vi "Handle.vi"(7 "Event jettl in":refnum<class "Event Actor.lvclass">, 11 "Teardown State in":refnum<class "Teardown State.lvclass">) -> (2 "Destroy?":bool, 5 "Event jettl out":refnum<class "Event Actor.lvclass">)   [LabVIEW 2021, in "jettl.lvlib" / "Base Event jettl.lvlib" / "Teardown State.lvclass"]
uses:
  Teardown State.lvclass
  Actor/Event Actor/Event Actor.lvclass
  Teardown State.lvclass/Teardown State.ctl
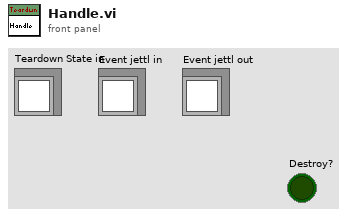
[diagram p1: front panel]
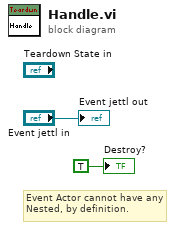
[diagram p0: block diagram]
diagram:
  # "Event Actor cannot have any Nested, by definition."
  "Destroy?" <- TRUE ("Destroy?")
  "Event jettl out" <- "Event jettl in"
